vi "Write Encoder Minimum Rate.vi"(8 "error in (no error)":errorcluster, 10 "Encoder Minimum Rate":dbl=100.0, 11 "DriveMotors in":refnum<class "DriveMotors.lvclass">) -> (0 "error out":errorcluster, 3 "DriveMotors out":refnum<class "DriveMotors.lvclass">)   [LabVIEW 2013, in "DriveMotors.lvclass"]
uses:
  DriveMotors.lvclass
  DriveMotors.lvclass/DriveMotors.ctl
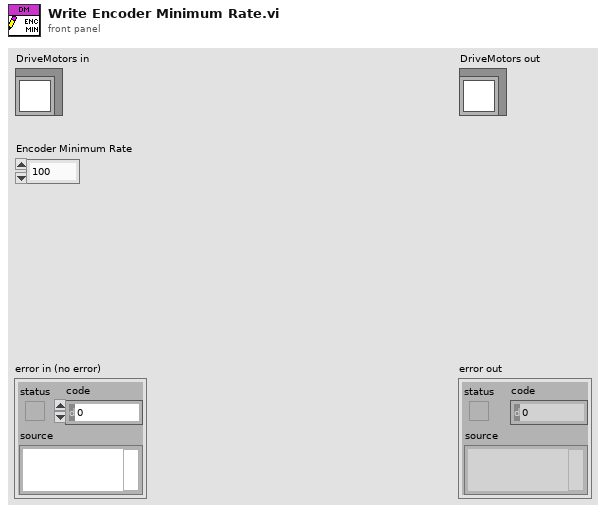
[diagram p1: front panel]
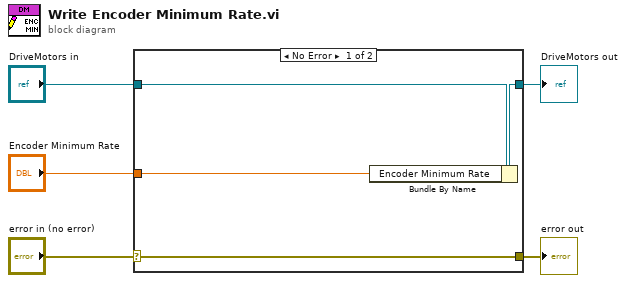
[diagram p0: block diagram]
diagram:
  n1 = case shown="No Error" "error in (no error)" {
    selector: "error in (no error)" -> [w9 w10]
    tunnel: [w9 w10] -> w4
    tunnel: [w7 w11] -> w2
    tunnel: "DriveMotors in" -> [w8 w11]
    tunnel: "Encoder Minimum Rate" -> [w6 _]
    frame No Error {
      n2 = Bundle By Name(cluster=w8, "Encoder Minimum Rate"=w6) -> (w7:refnum<class "DriveMotors.lvclass">)
    }
    frame Error {
    }
  }
  "error out" <- w4
  "DriveMotors out" <- w2
